vi "Add Discovered Object Instance (incoming).vi"(10 "discoverObjInstance":T1, 11 "hlaMap in":T2) -> (3 "hlaMap out":T2)   [LabVIEW 2019, in "HLA Custom Device Engine.lvlib"]
uses:
  HLA Custom Device Engine.lvlib
  _typedefs/RThlaMapHelpers.ctl
  _typedefs/map_in_interaction.ctl
  _typedefs/map_interaction_value.ctl
  _typedefs/map_attr_param_data.ctl
  _typedefs/map_object.ctl
  _typedefs/map_object_key.ctl
  _typedefs/map_object_value.ctl
  _typedefs/map_object_instance.ctl
  _typedefs/map_object_instance_value.ctl
  _typedefs/map_object_vs_instance.ctl
  _typedefs/map_out_vs_ch_instanceId.ctl
  _typedefs/map_out_vs_ch_objects.ctl
  _typedefs/map_out_vs_ch_objects_value.ctl
  _typedefs/map_out_vs_ch_interactIonClass.ctl
  _typedefs/discoverObjectInstance_type.ctl
  _Debug/VsDebugLibrary.lvlib
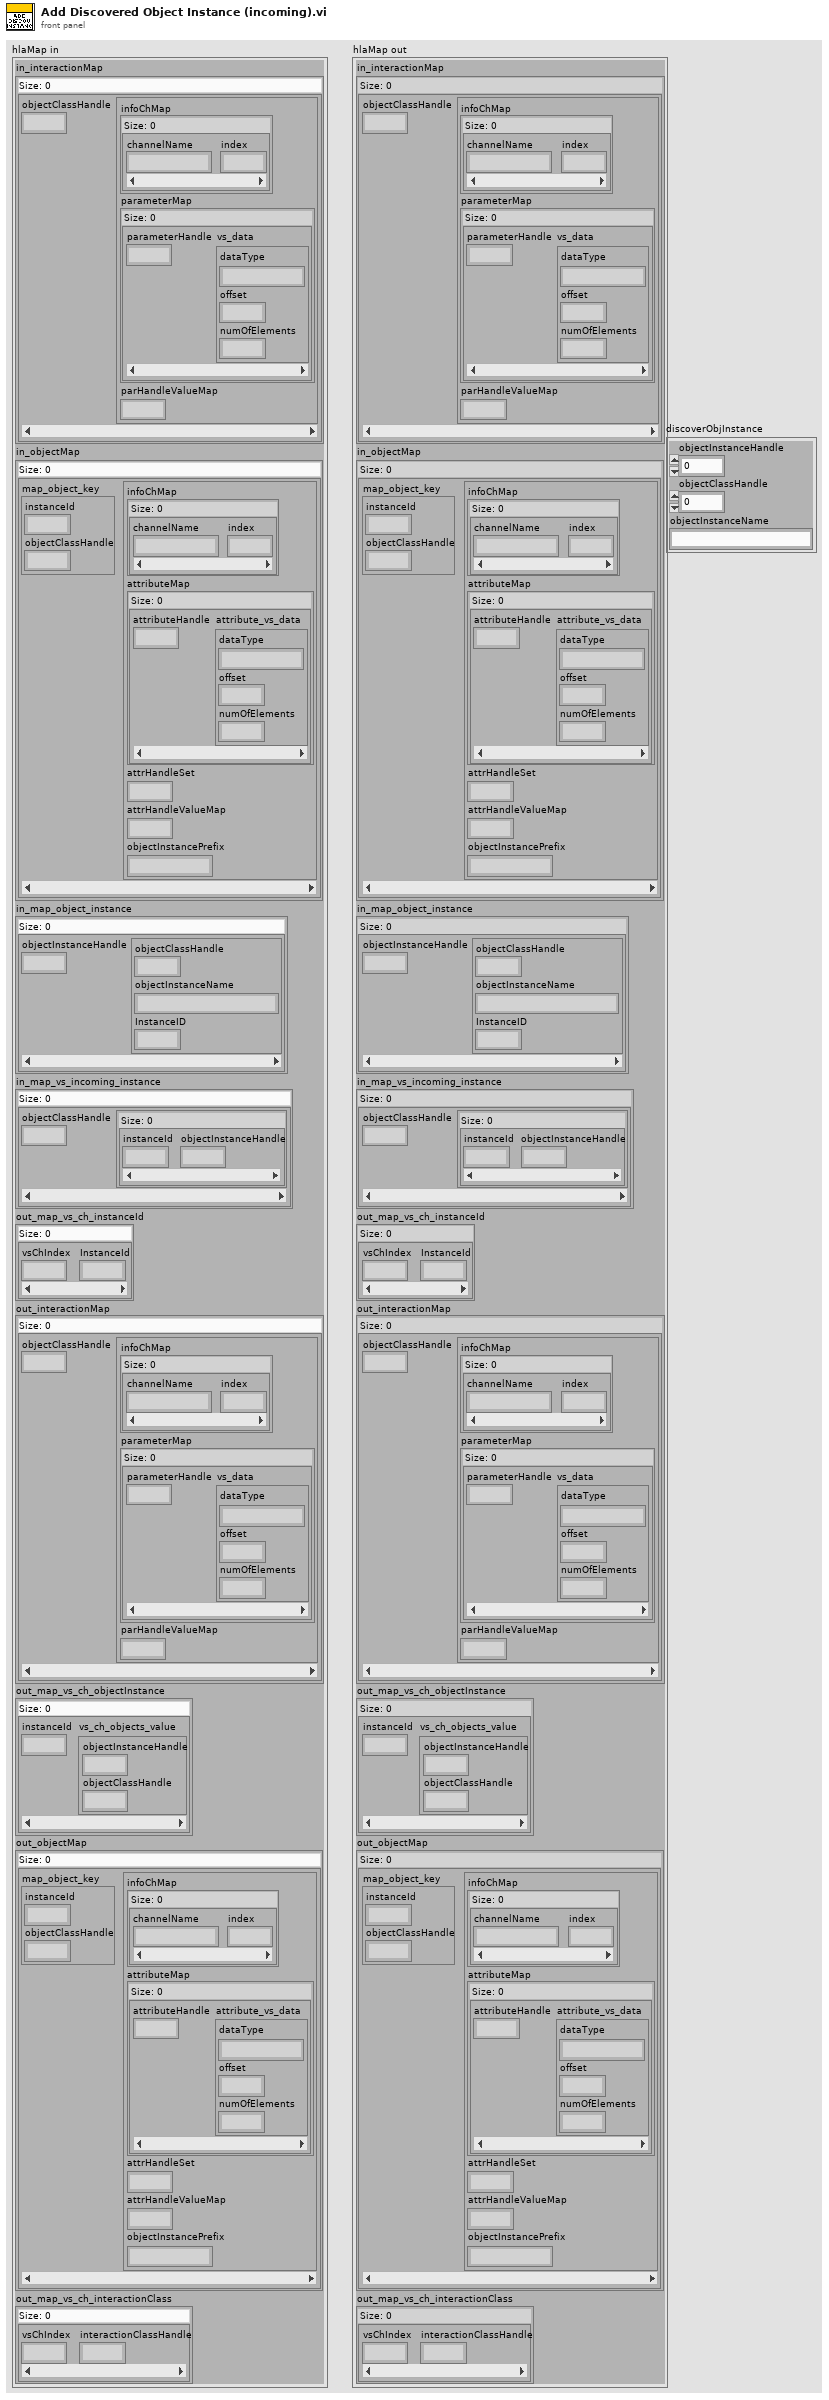
[diagram p1: front panel]
types:
  T1 = typedef "HLA Custom Device Engine.lvlib/discoverObjectInstance_type.ctl" = cluster{"objectInstanceHandle":u64, "objectClassHandle":u64, "objectInstanceName":string}
  T2 = typedef "HLA Custom Device Engine.lvlib/RThlaMapHelpers.ctl" = cluster{"in_interactionMap":T3, "in_objectMap":T6, "in_map_object_instance":T9, "in_map_vs_incoming_instance":T11, "out_map_vs_ch_instanceId":T12, "out_interactionMap":T3, "out_map_vs_ch_objectInstance":T13, "out_objectMap":T6, "out_map_vs_ch_interactionClass":T15}
  T3 = typedef "HLA Custom Device Engine.lvlib/map_in_interaction.ctl" = map{u64, T4}
  T4 = typedef "HLA Custom Device Engine.lvlib/map_interaction_value.ctl" = cluster{"infoChMap":map{string, i32}, "parameterMap":map{u64, T5}, "parHandleValueMap":u64}
  T5 = typedef "HLA Custom Device Engine.lvlib/map_attr_param_data.ctl" = cluster{"dataType":string, "offset":i32, "numOfElements":i32}
  T6 = typedef "HLA Custom Device Engine.lvlib/map_object.ctl" = map{T7, T8}
  T7 = typedef "HLA Custom Device Engine.lvlib/map_object_key.ctl" = cluster{"instanceId":i32, "objectClassHandle":u64}
  T8 = typedef "HLA Custom Device Engine.lvlib/map_object_value.ctl" = cluster{"infoChMap":map{string, i32}, "attributeMap":map{u64, T5}, "attrHandleSet":u64, "attrHandleValueMap":u64, "objectInstancePrefix":string}
  T9 = typedef "HLA Custom Device Engine.lvlib/map_object_instance.ctl" = map{u64, T10}
  T10 = typedef "HLA Custom Device Engine.lvlib/map_object_instance_value.ctl" = cluster{"objectClassHandle":u64, "objectInstanceName":string, "InstanceID":i32}
  T11 = typedef "HLA Custom Device Engine.lvlib/map_object_vs_instance.ctl" = map{u64, map{i32, u64}}
  T12 = typedef "HLA Custom Device Engine.lvlib/map_out_vs_ch_instanceId.ctl" = map{i32, i32}
  T13 = typedef "HLA Custom Device Engine.lvlib/map_out_vs_ch_objects.ctl" = map{i32, T14}
  T14 = typedef "HLA Custom Device Engine.lvlib/map_out_vs_ch_objects_value.ctl" = cluster{"objectInstanceHandle":u64, "objectClassHandle":u64}
  T15 = typedef "HLA Custom Device Engine.lvlib/map_out_vs_ch_interactIonClass.ctl" = map{i32, u64}
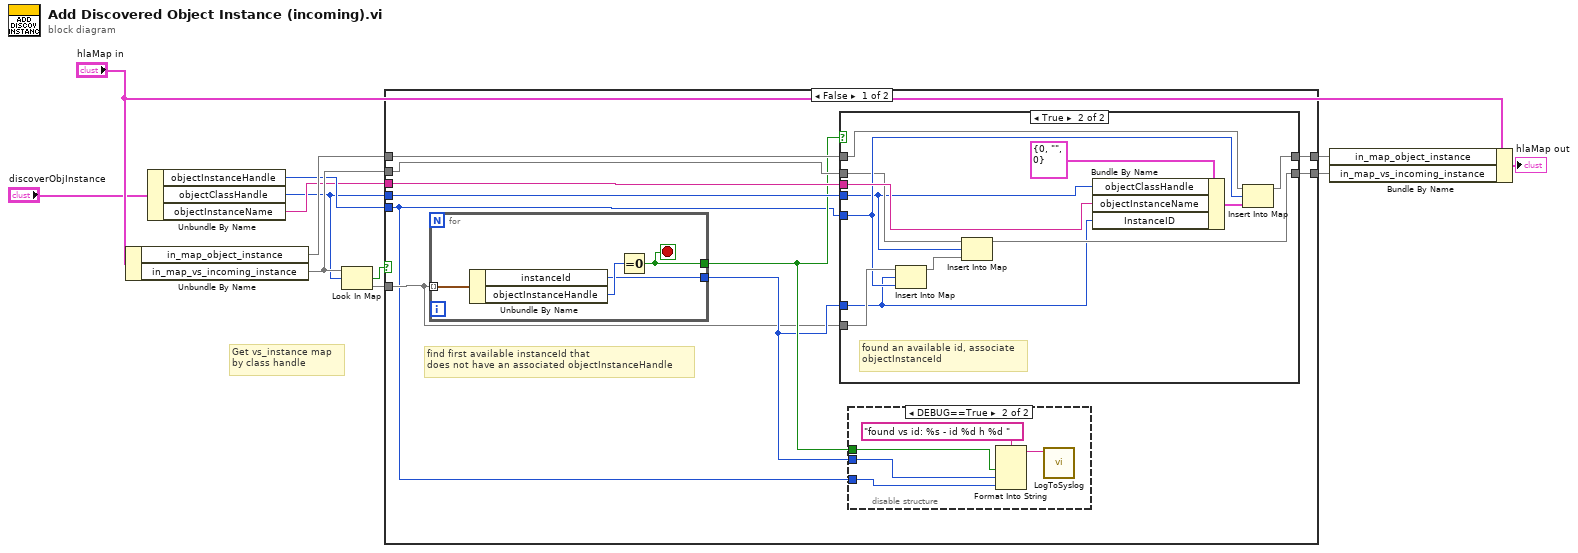
[diagram p0: block diagram]
diagram:
  # "Get vs_instance map \nby class handle"
  n1 = Unbundle By Name("hlaMap in") -> ("in_map_object_instance"=w10:T9, "in_map_vs_incoming_instance"=w8:T11)
  n2 = Unbundle By Name("discoverObjInstance") -> ("objectInstanceHandle"=w3:u64, "objectClassHandle"=w1:u64, "objectInstanceName"=w2:string)
  n3 = Look In Map(map=w8, key=w1) -> (key not found?=w7:bool, value=w12:map{i32, u64})  [unwired: 1 in]
  n4 = case shown="False" w7 {
    tunnel: w8 -> [w20 w47]
    tunnel: [w17 w47] -> w9
    tunnel: w10 -> [w19 w46]
    tunnel: [w18 w46] -> w11
    tunnel: w12 -> [w14 _]
    tunnel: w3 -> [w13 _]
    tunnel: w1 -> [w22 _]
    tunnel: w2 -> [w21 _]
    frame False {
      # "find first available instanceId that\ndoes not have an associated objectInstanceHandle"
      n5 = for {
        tunnel: w14 -> [w26] mode=indexing
        tunnel: [w24] -> w16
        tunnel: [w23] -> w15
        stop <- w24 stop-if-true
        n6 = Unbundle By Name(w26) -> ("instanceId"=w23:i32, "objectInstanceHandle"=w25:u64)
        n7 = Equal To 0?(x=w25) -> (x = 0?=w24:bool)
      }
      n8 = case shown="True" w16 {
        tunnel: w22 -> [_ w36]
        tunnel: w21 -> [_ w44]
        tunnel: w14 -> [_ w40]
        tunnel: w20 -> [w32 w38]
        tunnel: w19 -> [w33 w43]
        tunnel: [w33 w42] -> w18
        tunnel: w13 -> [_ w39]
        tunnel: [w32 w35] -> w17
        tunnel: w15 -> [_ w34]
        frame False {
        }
        frame True {
          # "found an available id, associate\nobjectInstanceId"
          n9 = Insert Into Map(map in=w40, key=w34, value=w39) -> (map out=w37:map{i32, u64})  [unwired: 2 out]
          n10 = Insert Into Map(map in=w38, key=w36, value=w37) -> (map out=w35:T11)  [unwired: 2 out]
          n11 = Bundle By Name(cluster=T10 {"objectClassHandle"=0, "objectInstanceName"="", "InstanceID"=0} ("value"), "objectClassHandle"=w36, "objectInstanceName"=w44, "InstanceID"=w34) -> (w41:T10)
          n12 = Insert Into Map(map in=w43, key=w39, value=w41) -> (map out=w42:T9)  [unwired: 2 out]
        }
      }
      n13 = disable-structure shown="DEBUG==True" {
        disable-tunnel: w15 -> [_ w28]
        disable-tunnel: w16 -> [_ w29]
        disable-tunnel: w13 -> [_ w27]
        frame condition #0 {
        }
        frame condition #1 (active) {
          n14 = Format Into String(format string="found vs id: %s - id %d h %d " ("message"), w29, w28, w27) -> (resulting string=w30:string)  [unwired: 2 in, 1 out]
          n15 = call "LogToSyslog.vi"("message"=w30) -> ()  [unwired: 9 in, 2 out]
        }
      }
    }
    frame True {
    }
  }
  n16 = Bundle By Name(cluster="hlaMap in", "in_map_object_instance"=w11, "in_map_vs_incoming_instance"=w9) -> (→"hlaMap out":T2)
